vi "MFCselection.vi"(5 "MFCsIn":T1[](array[typedef]), 6 "MdotMin":dbl=nan, 7 "MdotMax":dbl=nan, 9 "Mdot":dbl) -> (0 "OffCentre":dbl, 1 "errorMessage":string, 2 "nMFCs":i32, 4 "MFCsOut":T1[](array[typedef]))   [LabVIEW 2016]
uses:
  MFCdescription.ctl
  MFCcapability.ctl
  ComboRange.ctl
  MFCselectionData.ctl
  SelectionStages.ctl
panel:
  in  "Tab Control":enum32{"I/O", "Page 2", "PrivateData"}(tab)
  out "SuggestedRange":T3
  out "Array":T4[](array[typedef])
  out "Loops":i32
  out "Cluster":T5
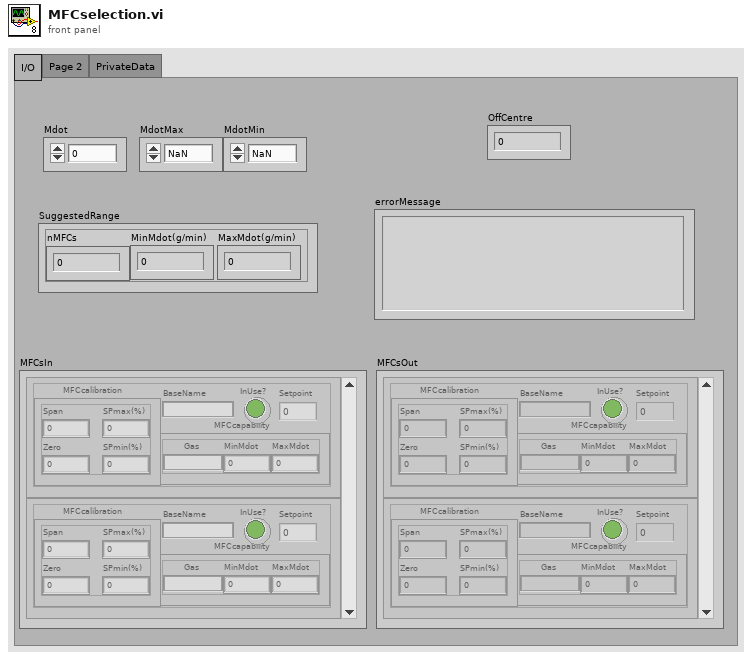
[diagram p1: front panel]
types:
  T1 = typedef "MFCdescription.ctl" = cluster{"BaseName":string, "MFCcalibration":cluster{"Span":dbl, "Zero":dbl, "SPmin(%)":dbl, "SPmax(%)":dbl}, "MFCcapability":T2, "InUse?":bool, "Setpoint":dbl}
  T2 = typedef "MFCcapability.ctl" = cluster{"Gas":string, "MinMdot":dbl, "MaxMdot":dbl}
  T3 = typedef "ComboRange.ctl" = cluster{"nMFCs":i32, "MinMdot(g/min)":dbl, "MaxMdot(g/min)":dbl}
  T4 = typedef "SelectionStages.ctl" = enum16{"Initialise", "HaveLimits?", "CurrentComboRange?", "GetAllCombos", "ExtractViableCombos", "EvaluateViableCombos", "WhatNext?", "ErrorReport", "FinalOutput"}
  T5 = typedef "MFCselectionData.ctl" = cluster{"MFCs":T1[], "Combos":T1[][], "Ranges":T3[], "MeritArray":dbl[], "SuggestedRange":T3, "suggestedCombo":T1[], "Merit":dbl, "nMFCs":i32, "OffCentreArray":dbl[], "OffCentre":dbl, "OverallMinMdot(g/min)":dbl, "OverallMaxMdot(g/min)":dbl}
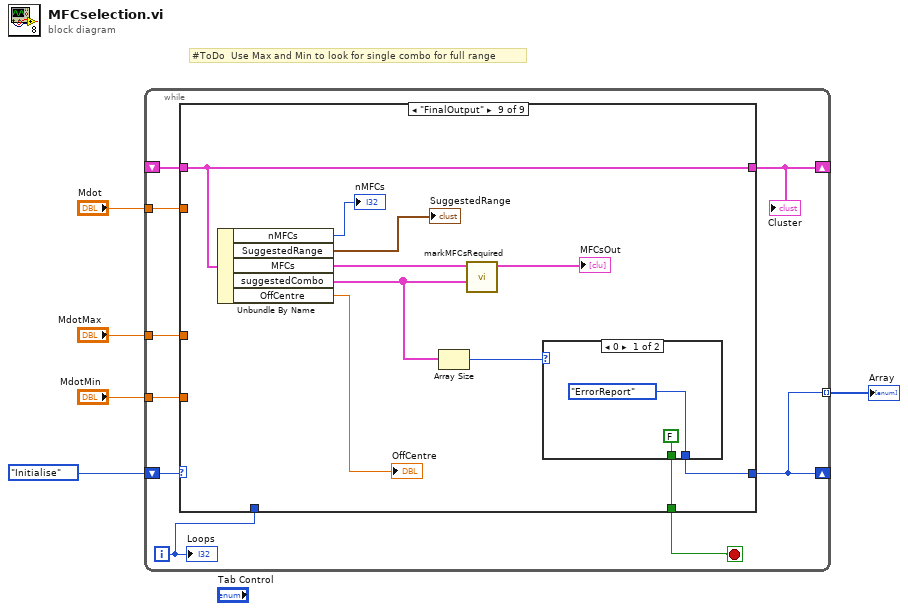
[diagram p0: block diagram]
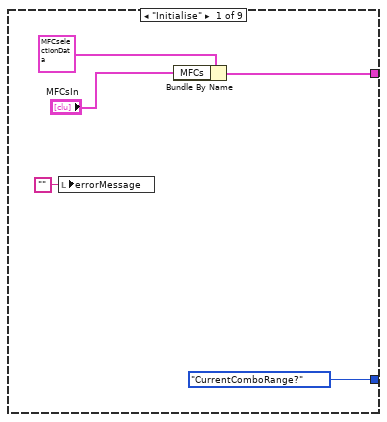
[diagram p2: hidden frame]
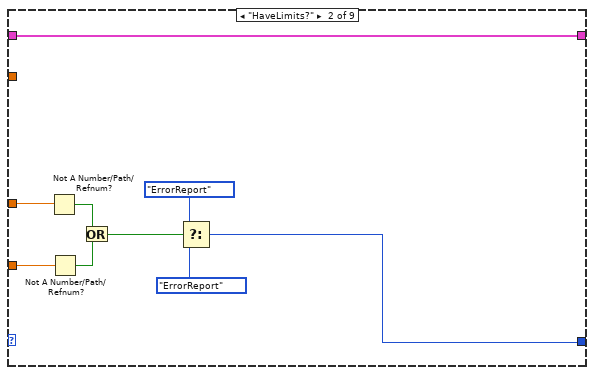
[diagram p3: hidden frame]
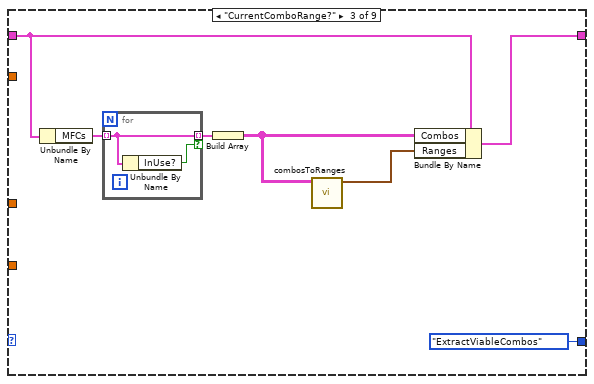
[diagram p4: hidden frame]
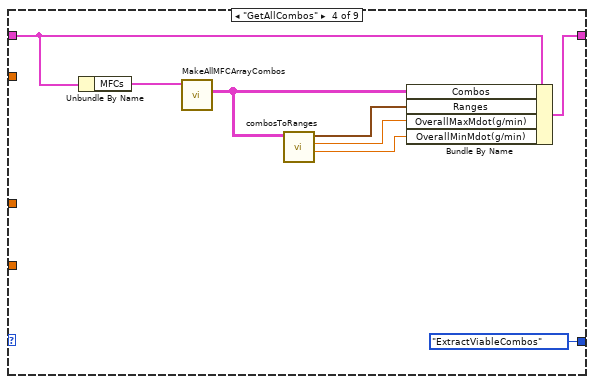
[diagram p5: hidden frame]
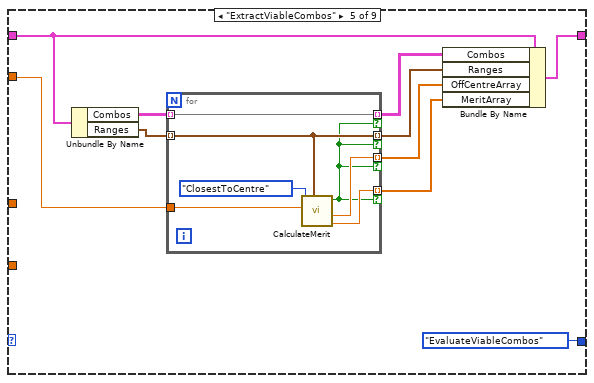
[diagram p6: hidden frame]
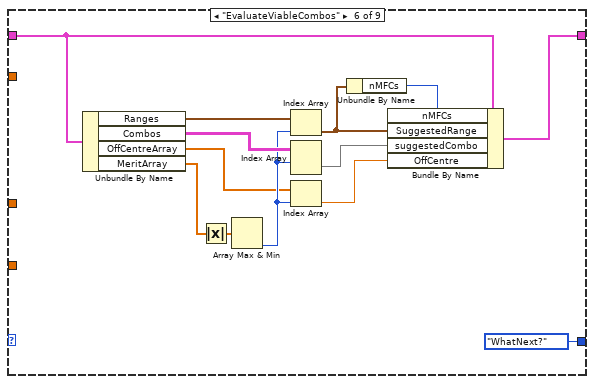
[diagram p7: hidden frame]
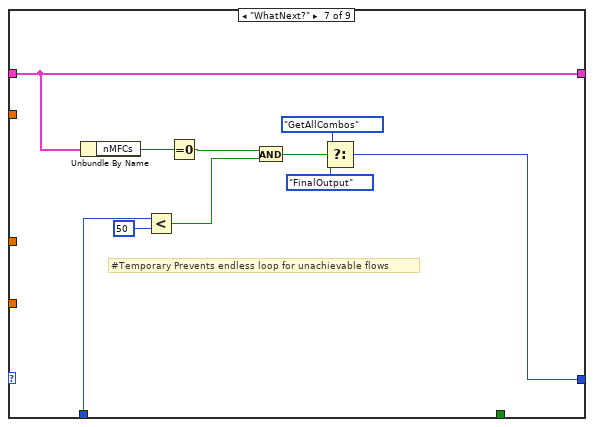
[diagram p8: hidden frame]
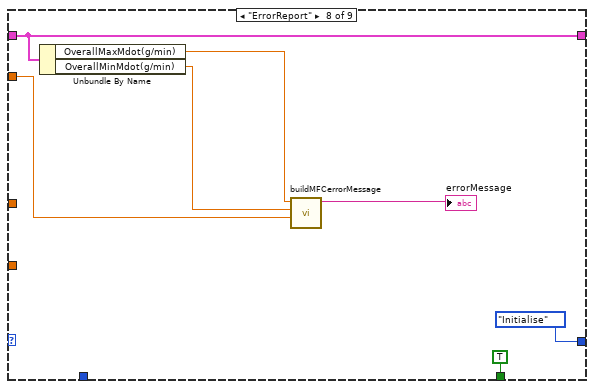
[diagram p9: hidden frame]
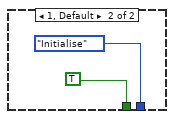
[diagram p10: hidden frame]
diagram:
  # "#ToDo  Use Max and Min to look for single combo for full range"
  n1 = while {
    shift-right: [w7] -> _
    shift-left: SelectionStages."Initialise" -> [w8]
    tunnel: "MdotMax" -> [w14]
    tunnel: "MdotMin" -> [w13]
    tunnel: "Mdot" -> [w12]
    shift-right: [w10] -> _
    shift-left: _ -> [w9]
    tunnel: [w7] -> w1 mode=indexing
    i -> [w6]
    stop <- w11 stop-if-true
    n2 = case shown="\"FinalOutput\"" w8 {
      tunnel: w14 -> [_ w28 _ _ _ _ _ _ _]
      tunnel: w13 -> [_ w27 _ _ _ _ _ _ _]
      tunnel: [SelectionStages."CurrentComboRange?" w22 SelectionStages."ExtractViableCombos" SelectionStages."ExtractViableCombos" SelectionStages."EvaluateViableCombos" SelectionStages."WhatNext?" w80 SelectionStages."Initialise" w98] -> w7
      tunnel: w12 -> [_ _ _ _ w54 _ _ w89 _]
      tunnel: [_ _ _ _ _ _ _ TRUE w99] -> w11
      tunnel: [w17 w20 w34 w43 w51 w65 w84 w90 w102] -> w10
      tunnel: w9 -> [_ w20 w31 w44 w52 w66 w84 w90 w102]
      tunnel: w6 -> [_ _ _ _ _ _ w79 _ _]
      frame "Initialise" {
        n3 = local write "errorMessage"("") -> ()
        n4 = Bundle By Name(cluster=T5 {"MFCs"=[], "Combos"=[], "Ranges"=[], "MeritArray"=[], "SuggestedRange"={"nMFCs"=0, "MinMdot(g/min)"=0.0, "MaxMdot(g/min)"=0.0}, "suggestedCombo"=[], "Merit"=0.0, "nMFCs"=0, "OffCentreArray"=[], "OffCentre"=0.0, "OverallMinMdot(g/min)"=0.0, "OverallMaxMdot(g/min)"=0.0}, "MFCs"="MFCsIn") -> (w17:T5)
      }
      frame "HaveLimits?" {
        n5 = Not A Number/Path/Refnum?(number/path/refnum=w28) -> (NaN/Path/Refnum?=w26:bool)
        n6 = Not A Number/Path/Refnum?(number/path/refnum=w27) -> (NaN/Path/Refnum?=w25:bool)
        n7 = Or(x=w26, y=w25) -> (x .or. y?=w24:bool)
        n8 = Select(t=SelectionStages."ErrorReport", s=w24, f=SelectionStages."ErrorReport") -> (s? t:f=w22:T4)
      }
      frame "CurrentComboRange?" {
        n9 = Unbundle By Name(w31) -> ("MFCs"=w30:T1[])
        n10 = for {
          tunnel: w30 -> [w37] mode=indexing
          tunnel: [w37] -> w29 mode=indexing if=w36
          n11 = Unbundle By Name(w37) -> ("InUse?"=w36:bool)
        }
        n12 = Build Array(w29) -> (w33:T1[][])
        n13 = call "combosToRanges.vi"("combosIn"=w33) -> ("rangesOut"=w35:T3[])  [unwired: 8 in, 2 out]
        n14 = Bundle By Name(cluster=w31, "Combos"=w33, "Ranges"=w35) -> (w34:T5)
      }
      frame "GetAllCombos" {
        n15 = Unbundle By Name(w44) -> ("MFCs"=w45:T1[])
        n16 = call "MakeAllMFCArrayCombos.vi"("EvaluatedMFCs"=w45) -> ("EveryCombination"=w42:T1[][])  [unwired: 10 in]
        n17 = call "combosToRanges.vi"("combosIn"=w42) -> ("OverallMinMdot(g/min)"=w38:dbl, "OverallMaxMdot(g/min)"=w39:dbl, "rangesOut"=w41:T3[])  [unwired: 8 in]
        n18 = Bundle By Name(cluster=w44, "Combos"=w42, "Ranges"=w41, "OverallMaxMdot(g/min)"=w39, "OverallMinMdot(g/min)"=w38) -> (w43:T5)
      }
      frame "ExtractViableCombos" {
        n19 = Unbundle By Name(w52) -> ("Combos"=w53:T1[][], "Ranges"=w55:T3[])
        n20 = for {
          tunnel: w55 -> [w60] mode=indexing
          tunnel: w54 -> [w61]
          tunnel: [w62] -> w50 mode=indexing if=w57
          tunnel: w53 -> [w62] mode=indexing
          tunnel: [w60] -> w49 mode=indexing if=w57
          tunnel: [w59] -> w47 mode=indexing if=w57
          tunnel: [w58] -> w46 mode=indexing if=w57
          n21 = call "CalculateMerit.vi"("RangeInfo"=w60, "Target"=w61, "MeritMeasure"=enum16{"MinMFCs", "ClosestToCentre", "Weighted"}."ClosestToCentre") -> ("Merit (smaller is better)"=w59:dbl, "OffsetFromCentre"=w58:dbl, "In Range?"=w57:bool)  [unwired: 5 in, 1 out]
        }
        n22 = Bundle By Name(cluster=w52, "Combos"=w50, "Ranges"=w49, "OffCentreArray"=w46, "MeritArray"=w47) -> (w51:T5)
      }
      frame "EvaluateViableCombos" {
        n23 = Unbundle By Name(w66) -> ("Ranges"=w74:T3[], "Combos"=w75:T1[][], "OffCentreArray"=w63:dbl[], "MeritArray"=w64:dbl[])
        n24 = Absolute Value(x=w64) -> (abs(x)=w73:dbl[])
        n25 = Array Max & Min(array=w73) -> (min index (indices)=w72:i32)  [unwired: 3 out]
        n26 = Index Array(array=w74, index=w72) -> (element=w69:T3)
        n27 = Index Array(array=w75, index (row)=w72) -> (element=w68:T1[])  [unwired: 1 in]
        n28 = Index Array(array=w63, index=w72) -> (element=w67:dbl)
        n29 = Unbundle By Name(w69) -> ("nMFCs"=w70:i32)
        n30 = Bundle By Name(cluster=w66, "nMFCs"=w70, "SuggestedRange"=w69, "suggestedCombo"=w68, "OffCentre"=w67) -> (w65:T5)
      }
      frame "WhatNext?" {
        # "#Temporary Prevents endless loop for unachievable flows"
        n31 = Unbundle By Name(w84) -> ("nMFCs"=w85:i32)
        n32 = Less?(x=w79, y=50) -> (x < y?=w76:bool)
        n33 = Equal To 0?(x=w85) -> (x = 0?=w83:bool)
        n34 = And(x=w83, y=w76) -> (x .and. y?=w77:bool)
        n35 = Select(t=SelectionStages."GetAllCombos", s=w77, f=SelectionStages."FinalOutput") -> (s? t:f=w80:T4)
      }
      frame "ErrorReport" {
        n36 = Unbundle By Name(w90) -> ("OverallMaxMdot(g/min)"=w88:dbl, "OverallMinMdot(g/min)"=w87:dbl)
        n37 = call "buildMFCerrorMessage.vi"("Mdot"=w89, "OverallMinMdot(g/min)"=w87, "OverallMaxMdot(g/min)"=w88) -> ("errorMessage"=→"errorMessage":string)  [unwired: 8 in]
      }
      frame "FinalOutput" {
        n38 = Unbundle By Name(w102) -> ("nMFCs"=→"nMFCs":i32, "SuggestedRange"=→"SuggestedRange":T3, "MFCs"=w96:T1[], "suggestedCombo"=w94:T1[], "OffCentre"=→"OffCentre":dbl)
        n39 = Array Size(array=w94) -> (size(s)=w93:i32)
        n40 = call "markMFCsRequired.vi"("suggestedCombo"=w94, "MFCsIn"=w96) -> ("MFCsOut"=→"MFCsOut":T1[])  [unwired: 9 in]
        n41 = case shown="0" w93 {
          tunnel: [FALSE TRUE] -> w99
          tunnel: [SelectionStages."ErrorReport" SelectionStages."Initialise"] -> w98
          frame 0 {
          }
          frame 1, Default {
          }
        }
      }
    }
    "Cluster" <- w10
    "Loops" <- w6
  }
  "Array" <- w1
